vi "WritePanelData_test_subpanelscorrect.vi"(8 "error in (no error)":errorcluster, 11 "Maui.Test.DefaultDirectory in":refnum<class "Maui.Test.DefaultDirectory.lvclass">) -> (0 "error out":errorcluster, 3 "Maui.Test.DefaultDirectory out":refnum<class "Maui.Test.DefaultDirectory.lvclass">)   [LabVIEW 2019, in "Maui.Test.DefaultDirectory.lvclass"]
uses:
  Maui.Test.DefaultDirectory.lvclass
  C:/Users/Patrick/Documents/GitHub/MAUI-Engine/lvsrc/Maui 1.0/SMO.UI.MAUI/SMO.UI.MAUI.lvclass
  Maui.Test.DefaultDirectory.lvclass/Maui.Test.DefaultDirectory.ctl
  <vilib>/addons/_JKI Toolkits/Caraya/classes/Assert/Assert Equal Value_Variant.vi
  lvsrc/Maui 1.0/SMO.UI.MAUI/SMO.UI.MAUI.lvclass
  <userlib>/LevyLab/Embedded UI/SMO.UI.Embedded/SMO.UI.Embedded.lvclass
  <vilib>/addons/_JKI Toolkits/Caraya/classes/Assert/Assert.lvclass
  <vilib>/addons/_JKI Toolkits/Caraya/classes/Test/Test.lvclass
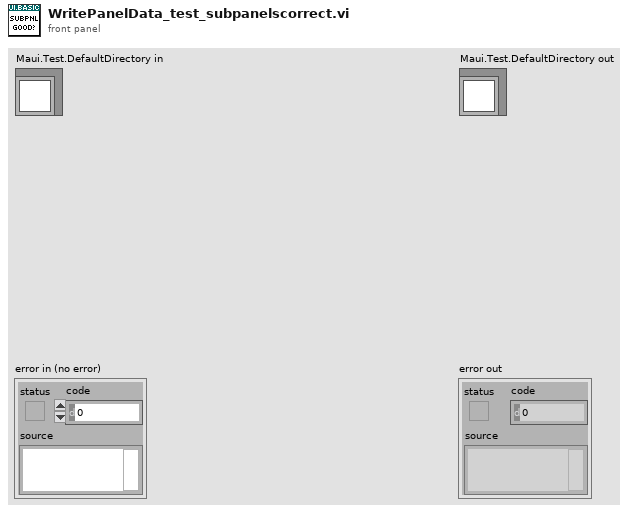
[diagram p1: front panel]
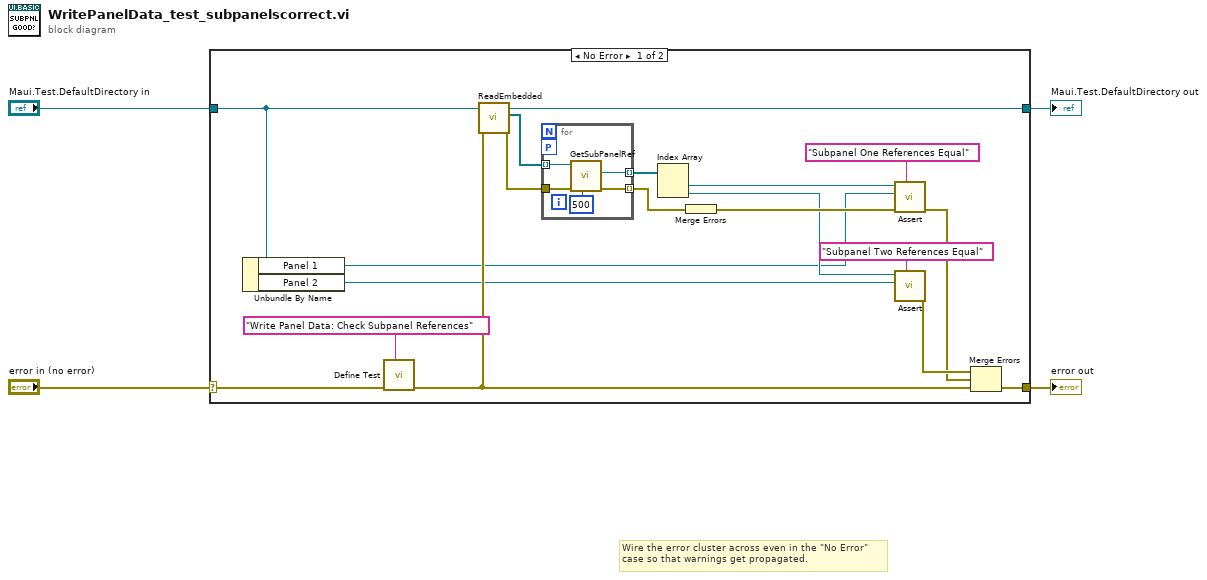
[diagram p0: block diagram]
diagram:
  # "Wire the error cluster across even in the \"No Error\"\ncase so that warnings get propagated."
  n1 = case shown="No Error" "error in (no error)" {
    selector: "error in (no error)" -> [w13 w28]
    tunnel: [w8 w29] -> w2
    tunnel: "Maui.Test.DefaultDirectory in" -> [w8 w29]
    tunnel: [w15 w28] -> w1
    frame No Error {
      n2 = Unbundle By Name(w8) -> ("Panel 1"=w7:refnum<vi>, "Panel 2"=w6:refnum<vi>)
      n3 = call <vilib>:"Define Test.vi"("error in (no error)"=w13, "Label (VI Title)"="Write Panel Data: Check Subpanel References") -> ("error out"=w12:errorcluster)  [unwired: 9 in]
      n4 = call "ReadEmbedded.vi"("error in (no error)"=w12, "MAUI in"=w8) -> ("error out"=w18:errorcluster, "Subpanels"=w22:refnum<class "SMO.UI.Embedded.lvclass">[])  [unwired: 7 in, 1 out]
      n5 = for {
        tunnel: w22 -> [w27] mode=indexing
        tunnel: [w26] -> w21 mode=indexing
        tunnel: [w24] -> w17 mode=indexing
        workers-P: _ -> [_]
        tunnel: w18 -> [w23]
        n6 = call <userlib>:"GetSubPanelRef.vi"("timeout in ms (-1)"=500, "error in (no error)"=w23, "EmbeddedSMO in"=w27) -> ("error out"=w24:errorcluster, "SubPanelReference"=w26:refnum<vi>)  [unwired: 6 in, 1 out]
      }
      n7 = Index Array(array=w21) -> (element #1=w19:refnum<vi>, element #2=w11:refnum<vi>)  [unwired: 2 in]
      n8 = Merge Errors(w17) -> (w16:errorcluster)
      n9 = call-poly <vilib>:"Assert.vi"("Label"="Subpanel One References Equal" ("Label (VI Title)"), "error in (no error)"=w16, "Y"=w7, "X"=w19) -> ("error out"=w9:errorcluster)  [unwired: 7 in]
      n10 = call-poly <vilib>:"Assert.vi"("Label"="Subpanel Two References Equal" ("Label (VI Title)"), "Y"=w6, "X"=w11) -> ("error out"=w10:errorcluster)  [unwired: 8 in]
      n11 = Merge Errors(w10, w9, w12) -> (w15:errorcluster)
    }
    frame Error {
    }
  }
  "error out" <- w1
  "Maui.Test.DefaultDirectory out" <- w2
